vi "NISE.remote.Close Property.vi"(0 "SLSC Remote in":refnum<class "SLSC Interface.lvclass">, 5 "property":refnum<k21>, 11 "error in (no error)":errorcluster) -> (4 "SLSC Remote out":refnum<class "SLSC Interface.lvclass">, 15 "error out":errorcluster)   [LabVIEW 2016, in "SLSC Interface.lvclass"]
uses:
  SLSC Interface Class/SLSC Interface.lvclass
  SLSC Interface Class/SLSC Interface.lvclass/SLSC Interface.ctl
  SLSC Interface Class/NISE.Read client handle.vi
  SLSC Interface Class/NISE.Read URL.vi
  SLSC Interface Class/NISE.Read session.vi
  <vilib>/NI/JSON Support for LabVIEW/JSON Value/New JSON Value/New JSON ({String}).vi
  <vilib>/NI/NI JSONRPC Server Framework/Classes/Server/server.Format Client Request (Auto-Increment).vi
  <vilib>/httpClient/POSTBuffer.vi
  <vilib>/httpClient/LabVIEWHTTPClient.lvlib
  <vilib>/NI/NI JSONRPC Server Framework/Classes/Server/JSONRPC Server.lvclass
  <vilib>/NI/JSON Support for LabVIEW/JSON Value/JSON Value.lvclass
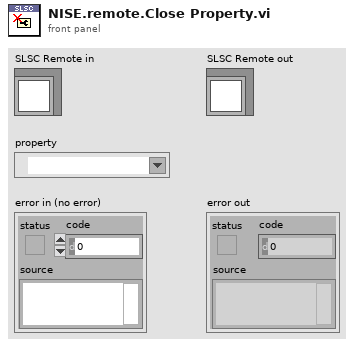
[diagram p1: front panel]
types:
  T1 = typedef "LabVIEWHTTPClient.lvlib/ClientHandle.ctl" = refnum<k1>
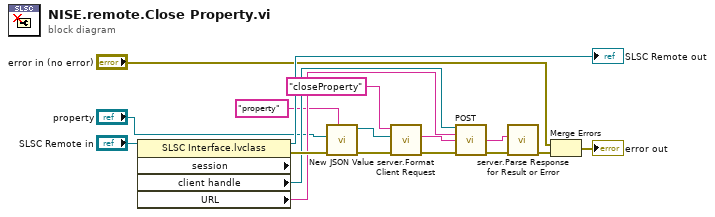
[diagram p0: block diagram]
diagram:
  n1 = property class="SLSC Interface.lvclass" props=["session", "client handle", "URL"](reference="SLSC Remote in") -> (reference out=→"SLSC Remote out":refnum<class "SLSC Interface.lvclass">, error out=w15:errorcluster, "client handle"=w11:T1, "URL"=w10:string)  [unwired: 1 in, 1 out]
  n2 = call-poly <vilib>:"New JSON Value.vi"("key"="property" ("Name"), "error in (no error)"=w15, "value"="property") -> ("error out"=w14:errorcluster, "JSON Value out"=w1:refnum<class "JSON Value.lvclass">)  [unwired: 7 in]
  n3 = call-poly <vilib>:"server.Format Client Request.vi"("error in (no error)"=w14, "JSON Value in"=w1, "method"="closeProperty") -> ("error out"=w9:errorcluster, "Request String"=w12:string)  [unwired: 7 in]
  n4 = call-poly <vilib>:"POST.vi"("client handle"=w11, "url"=w10, "buffer"=w12, "error in (no error)"=w9) -> ("body"=w8:string, "error out"=w7:errorcluster)  [unwired: 8 in, 2 out]
  n5 = call <vilib>:"server.Parse Response for Result or Error.vi"("error in"=w7, "Response String In"=w8) -> ("error out"=w6:errorcluster)  [unwired: 7 in, 2 out]
  n6 = Merge Errors("error in (no error)", w6) -> (→"error out":errorcluster)
